vi "Find all dependencies in a folder or folders.vi"() -> ()   [LabVIEW 2013]
doc: "This .vi will analyze the .vi's in the selected folder/paths for dependencies outside the project. This utility first loads all of the vi's in the input list into memory. It then computes a dependency list strictly comparing the .vi's in memory to the .vi's in the project. \n\nTherefore, if code is conditionally disabled, those .vi's will not make the list, as long as they are not in memory. To make sure they are not in memory, close all of those .vi's and their callers."
uses:
  <vilib>/Utility/miscctls.llb/LVRowAndColumnUnsignedTypeDef.ctl
panel:
  out "Dependencies":string[][](table)=[["HHMI - Beam size info cluster.ctl", "\\Quartz LV8.6 VIs\\Motion\\Beam Size\\Low level\\Typedefs\\", "HHMI - Beam size spreadsheet string to cluster converter.vi", "\\Common LV8.6 VIs\\Alignment\\Calibration\\Cal Files\\Load and Save\\"], ["HHMI - Beam sizes enum.ctl", "\\Quartz LV8.6 VIs\\Motion\\Beam Size\\Low level\\Typedefs\\", "HHMI - Beam size spreadsheet string to cluster converter.vi", "\\Common LV8.6 VIs\\Alignment\\Calibration\\Cal Files\\Load and Save\\"], ["HHMI - Frame Timing cluster.ctl", "\\Quartz LV8.6 VIs\\Scan\\Typedefs\\", "HHMI - Time elasped.vi", "\\Common LV8.6 VIs\\Utilities\\"], ["HHMI - Overlap size Cluster.ctl", "\\Quartz LV8.6 VIs\\Adaptive Optics\\Typedefs\\", "HHMI - Convert SLM Settings to Overlap sizes Cluster.vi", "\\Common LV8.6 VIs\\SLM\\Rear Pupil\\"], ["HHMI - Pixel Parameters cluster.ctl", "\\Quartz LV8.6 VIs\\Scan\\Waveform\\Typedefs\\", "HHMI - Calibrated montage image references ID generator.vi", "\\Common LV8.6 VIs\\Alignment\\Functional Globals\\"], ["HHMI - Time control enum.ctl", "\\Quartz LV8.6 VIs\\Scan\\Typedefs\\", "HHMI - Prepare for alignment to active SLM regions.vi", "\\Common LV8.6 VIs\\Alignment\\"], ["HHMI - Waveform Configuration cluster.ctl", "\\Quartz LV8.6 VIs\\Scan\\Waveform\\Typedefs\\", "HHMI - Calibrated montage image references ID generator.vi", "\\Common LV8.6 VIs\\Alignment\\Functional Globals\\"], ["HHMI - Waveform Type enum.ctl", "\\Quartz LV8.6 VIs\\Scan\\Waveform\\Typedefs\\", "HHMI - Calibrated montage image references ID generator.vi", "\\Common LV8.6 VIs\\Alignment\\Functional Globals\\"]]
  in  "stop":bool
  in  "Open FP's of Parents?":bool
  in  "Parent paths to remove in Path column":i32=10
  in  "Include .ctl's":bool=TRUE
  in  "Include .vi's":bool=TRUE
  out "Current Project":string="Common"
  out "Progress":i32(slide)=525 scale=-1.0..2.0
  in  "Paths":path[](array[path])=[path "C:/Users/dmilkie/Documents/CTI/PROJECTS/HHMI/HHMI - Common/Common Project/Common LV8.6 VIs"]
  # "Warning : Parent VIs don't list static VI refs."
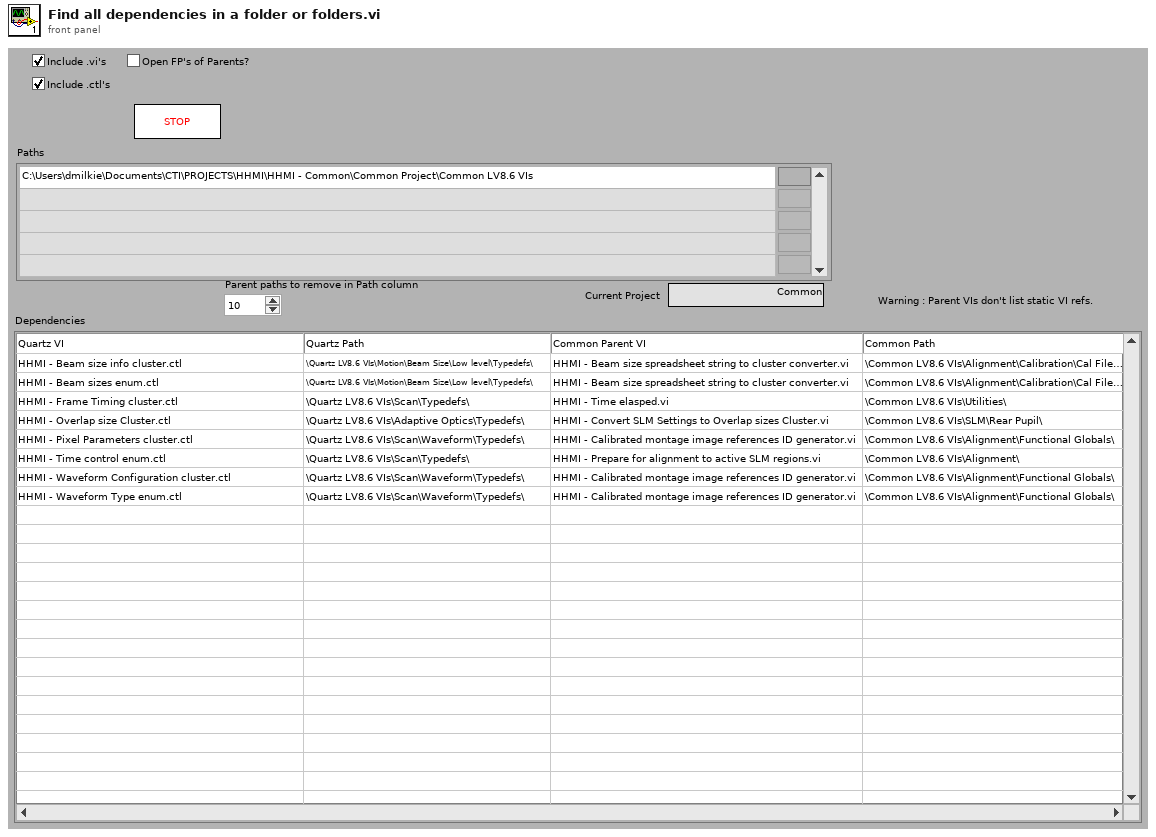
[diagram p1: front panel]
types:
  T1 = typedef "LVRowAndColumnUnsignedTypeDef.ctl" = cluster{"Row":u32, "Column":u32}
  T2 = typedef "Dependency cluster.ctl" = cluster{"VI name":string, "Path":path, "Parent project VI":string, "Parent path":path}
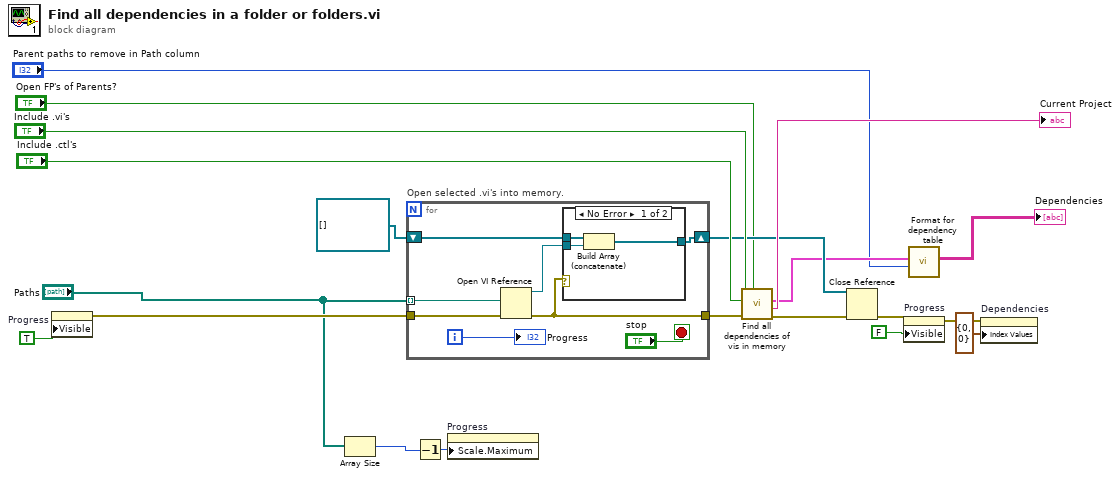
[diagram p0: block diagram]
diagram:
  n1 = property on="Progress" class="Slide (strict)"("Visible"=TRUE) -> (error out=w5:errorcluster)  [unwired: 2 in, 1 out]
  n2 = Array Size(array="Paths") -> (size(s)=w19:i32)
  n3 = for "Open selected .vi's into memory." {
    tunnel: "Paths" -> [w28] mode=indexing
    tunnel: [w27] -> w6
    tunnel: w5 -> [w22]
    shift-right: [w25] -> w13
    shift-left: refnum<vi>[] [] -> [w26]
    i -> [w24]
    stop <- "stop" stop-if-true
    n4 = Open VI Reference(vi path=w28, error in (no error)=w22) -> (vi reference=w23:refnum<vi>, error out=w27:errorcluster)  [unwired: 4 out]
    n5 = case shown="No Error" w27 {
      tunnel: w23 -> [w29 _]
      tunnel: w26 -> [w31 w32]
      tunnel: [w30 w32] -> w25
      frame No Error {
        n6 = Build Array (concatenate)(w31, w29) -> (w30:refnum<vi>[])
      }
      frame Error {
        # "Not a .vi or .ctl"
      }
    }
    "Progress" <- w24
  }
  n7 = Decrement(x=w19) -> (x-1=w15:i32)
  n8 = property on="Progress" class="Slide (strict)"("Scale.Maximum"=w15) -> ()  [unwired: 2 in, 2 out]
  n9 = call "Find all dependencies of vis in memory.vi"("Open FP's of Parents?"="Open FP's of Parents?", "error in"=w6, "Include .ctl's"="Include .ctl's", "Include .vi's"="Include .vi's") -> ("error out"=w12:errorcluster, "Project"=→"Current Project":string, "Dependencies"=w10:T2[])  [unwired: 5 out]
  n10 = Close Reference(reference=w13, error in (no error)=w12) -> (error out=w8:errorcluster)
  n11 = property on="Progress" class="Slide (strict)"(error in=w8, "Visible"=FALSE) -> (error out=w3:errorcluster)  [unwired: 1 in, 1 out]
  n12 = call "Format for dependency table.vi"("# of Parent paths to remove in Path column"="Parent paths to remove in Path column", "Dependencies"=w10) -> ("ItemNames"=→"Dependencies":string[][])  [unwired: 1 in, 4 out]
  n13 = property on="Dependencies" class="Tbl (strict)"(error in=w3, "Index Values"=T1 {"Row"=0, "Column"=0}) -> ()  [unwired: 1 in, 2 out]
